vi "RegisterCheck.vi"(8 "error in":errorcluster caption="错误输入", 9 "CMD2":string="AT+CGREG?", 10 "CMD1":string="AT+CREG?", 11 "COMIn":refnum<visa-resource-name>) -> (0 "error out":errorcluster caption="错误输出", 1 "反馈":string, 3 "Result":bool)   [LabVIEW 2013]
uses:
  C:/Program Files/National Instruments/LabVIEW 2013/examples/Instrument IO/Serial/support/Serial - Settings.ctl
  <vilib>/Instr/_visa.llb/VISA Flush IO Buffer Mask.ctl
  <vilib>/Instr/_visa.llb/VISA Configure Serial Port (Instr).vi
panel:
  out "CGREG响应":string
  out "CREG响应":string
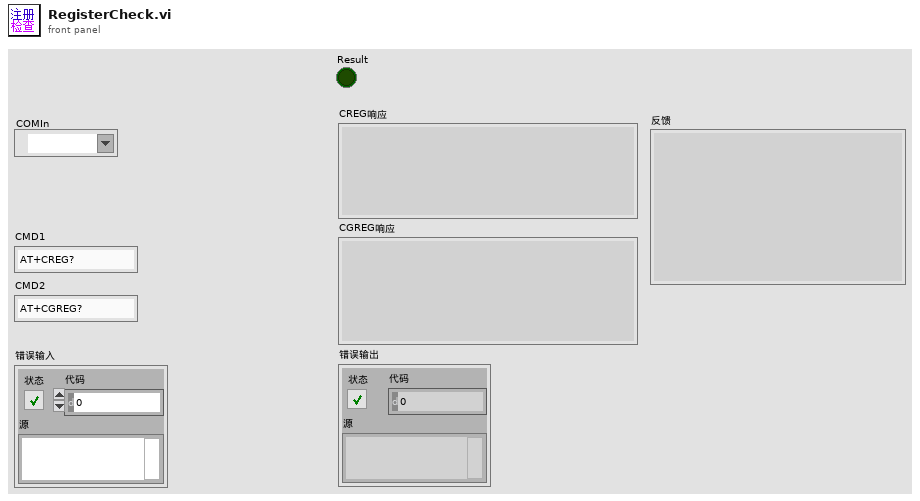
[diagram p1: front panel]
types:
  T1 = typedef "VISA Flush IO Buffer Mask.ctl" = u16
  T2 = typedef "Serial - Settings.ctl" = cluster{"波特率":u32, "数据比特":u16, "奇偶":enum16{"None", "Odd", "Even", "Mark", "Space"}, "停止位":u16, "流控制":u16}
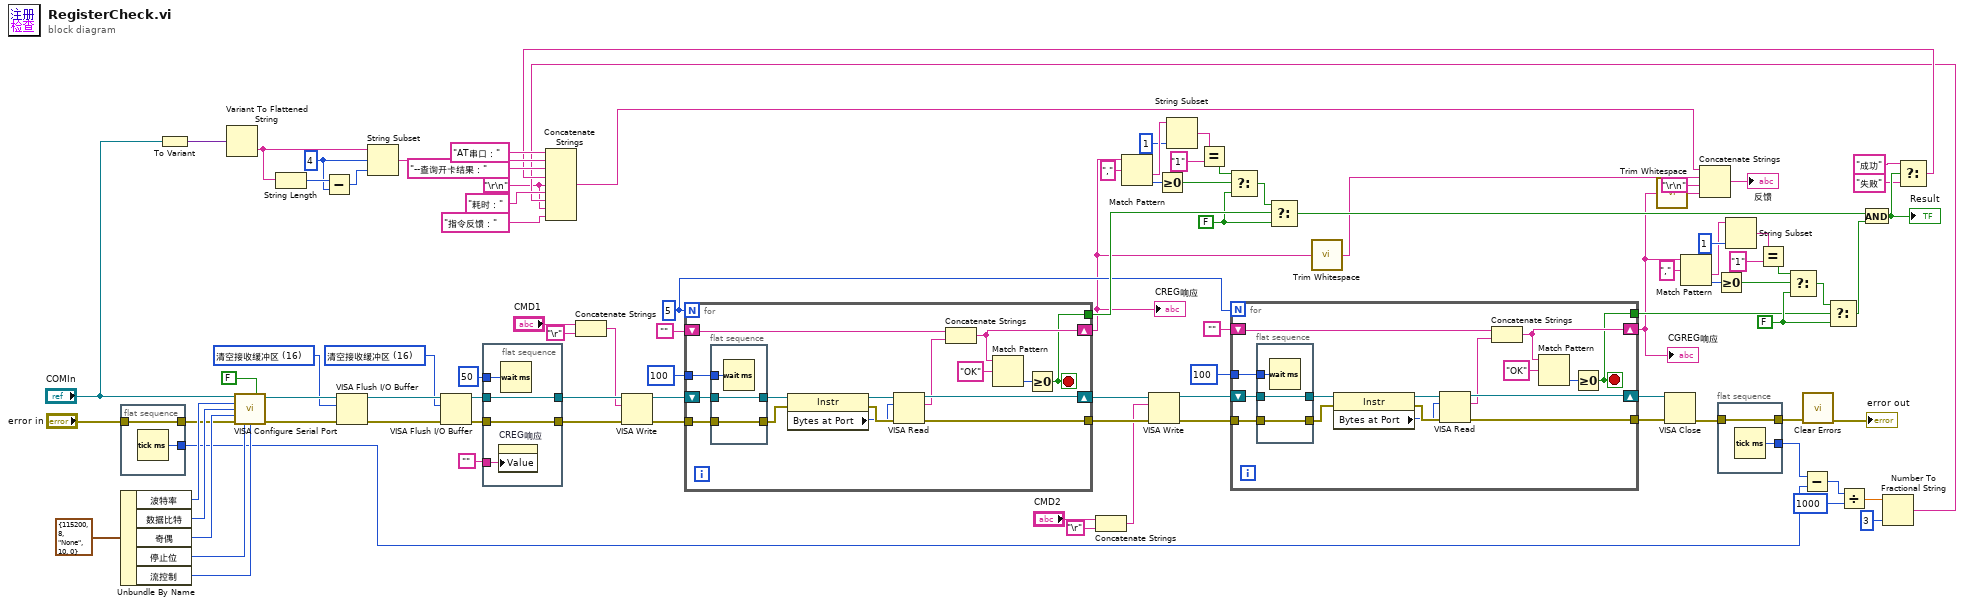
[diagram p0: block diagram]
diagram:
  w3 = "\r\n"
  w24 = 4
  w57 = FALSE
  w61 = FALSE
  w38 = 5
  w85 = T1 16 items=["清空接收缓冲区"=16, "向设备写入传输缓冲区"=32, "清空接收缓冲区（无I/O）"=64, "清空传输缓冲区"=128] ("Mask")
  w88 = T1 16 items=["清空接收缓冲区"=16, "向设备写入传输缓冲区"=32, "清空接收缓冲区（无I/O）"=64, "清空传输缓冲区"=128] ("Mask")
  n1 = flat-sequence {
    tunnel: [w99] -> w15
    tunnel: "error in" -> [w99]
    tunnel: [w98] -> w10
    frame #0 {
      n2 = Tick Count (ms)() -> (millisecond timer value=w98:u32)
    }
  }
  n3 = Unbundle By Name(T2 {"波特率"=115200, "数据比特"=8, "奇偶"=enum."None", "停止位"=10, "流控制"=0} ("串口设置")) -> ("波特率"=w96:u32, "数据比特"=w95:u16, "奇偶"=w94:enum16{"None", "Odd", "Even", "Mark", "Space"}, "停止位"=w93:u16, "流控制"=w92:u16)
  n4 = To Variant(anything="COMIn") -> (Variant=w28:variant)
  n5 = Variant To Flattened String(Variant=w28) -> (data string=w27:string)  [unwired: 1 out]
  n6 = call-poly "VISA Configure Serial Port"("VISA resource name"="COMIn", "Enable Termination\nChar (T)"=FALSE ("Enable Termination\nChar (T)"), "baud rate (9600)"=w96, "data bits (8)"=w95, "parity (0:none)"=w94, "error in (no error)"=w15, "stop bits (10: 1 bit)"=w93, "flow control (0:none)"=w92) -> ("VISA resource name out"=w90:refnum<visa-resource-name>, "error out"=w89:errorcluster)  [unwired: 6 in]
  n7 = String Length(string=w27) -> (length=w26:i32)
  n8 = Subtract(x=w26, y=w24) -> (x-y=w25:i32)
  n9 = VISA Flush I/O Buffer(VISA resource name=w90, mask (16)=w88, error in (no error)=w89) -> (VISA resource name out=w87:refnum<visa-resource-name>, error out=w86:errorcluster)
  n10 = String Subset(string=w27, offset (0)=w24, length (rest)=w25) -> (substring=w23:string)
  n11 = VISA Flush I/O Buffer(VISA resource name=w87, mask (16)=w85, error in (no error)=w86) -> (VISA resource name out=w84:refnum<visa-resource-name>, error out=w83:errorcluster)
  n12 = flat-sequence {
    tunnel: w84 -> [w102]
    tunnel: [w101] -> w80
    tunnel: w83 -> [w101]
    tunnel: 50 -> [w103]
    tunnel: [w102] -> w81
    tunnel: "" -> [w100]
    frame #0 {
      n13 = property on="CREG响应" class="Str"("Value"=w100) -> ()  [unwired: 2 in, 2 out]
      n14 = Wait (ms)(milliseconds to wait=w103) -> ()  [unwired: 1 out]
    }
  }
  n15 = Concatenate Strings("CMD1", "\r") -> (w78:string)
  n16 = VISA Write(VISA resource name=w81, write buffer=w78, error in (no error)=w80) -> (VISA resource name out=w76:refnum<visa-resource-name>, error out=w75:errorcluster)  [unwired: 1 out]
  n17 = for {
    N: w38 -> [_]
    shift-right: [w111] -> w46
    shift-left: w76 -> [w119]
    tunnel: w75 -> [w118]
    tunnel: 100 -> [w117]
    shift-right: [w107] -> w34
    shift-left: "" -> [w110]
    tunnel: [w108] -> w44
    tunnel: [w104] -> w63
    stop <- w104 stop-if-true
    n18 = flat-sequence {
      tunnel: w119 -> [w121]
      tunnel: w118 -> [w120]
      tunnel: w117 -> [w122]
      tunnel: [w121] -> w116
      tunnel: [w120] -> w115
      frame #0 {
        n19 = Wait (ms)(milliseconds to wait=w122) -> ()  [unwired: 1 out]
      }
    }
    n20 = property class="Instr"(reference=w116, error in=w115) -> (reference out=w112:refnum<visa-resource-name>, error out=w114:errorcluster, "Bytes at Port"=w113:u32)
    n21 = VISA Read(VISA resource name=w112, byte count=w113, error in (no error)=w114) -> (VISA resource name out=w111:refnum<visa-resource-name>, read buffer=w109:string, error out=w108:errorcluster)  [unwired: 1 out]
    n22 = Concatenate Strings(w110, w109) -> (w107:string)
    n23 = Match Pattern(string=w107, regular expression="OK" ("正则表达式")) -> (offset past match=w105:i32)  [unwired: 1 in, 3 out]
    n24 = Greater Or Equal To 0?(x=w105) -> (x >= 0?=w104:bool)
  }
  "CREG响应" <- w34
  n25 = Concatenate Strings("CMD2", "\r") -> (w39:string)
  n26 = Match Pattern(string=w34, regular expression="," ("正则表达式")) -> (after substring=w68:string, offset past match=w70:i32)  [unwired: 1 in, 2 out]
  n27 = VISA Write(VISA resource name=w46, write buffer=w39, error in (no error)=w44) -> (VISA resource name out=w45:refnum<visa-resource-name>, error out=w43:errorcluster)  [unwired: 1 out]
  n28 = Greater Or Equal To 0?(x=w70) -> (x >= 0?=w69:bool)
  n29 = String Subset(string=w68, length (rest)=1 ("长度（剩余）")) -> (substring=w66:string)  [unwired: 1 in]
  n30 = Equal?(x=w66, y="1") -> (x = y?=w64:bool)
  n31 = Select(t=w64, s=w69, f=w61) -> (s? t:f=w62:bool)
  n32 = for {
    N: w38 -> [_]
    shift-right: [w130] -> w60
    shift-left: w45 -> [w138]
    tunnel: w43 -> [w137]
    tunnel: 100 -> [w136]
    shift-right: [w126] -> w35
    shift-left: "" -> [w129]
    tunnel: [w127] -> w59
    tunnel: [w123] -> w47
    stop <- w123 stop-if-true
    n33 = flat-sequence {
      tunnel: w138 -> [w140]
      tunnel: w137 -> [w139]
      tunnel: w136 -> [w141]
      tunnel: [w140] -> w135
      tunnel: [w139] -> w134
      frame #0 {
        n34 = Wait (ms)(milliseconds to wait=w141) -> ()  [unwired: 1 out]
      }
    }
    n35 = property class="Instr"(reference=w135, error in=w134) -> (reference out=w131:refnum<visa-resource-name>, error out=w133:errorcluster, "Bytes at Port"=w132:u32)
    n36 = VISA Read(VISA resource name=w131, byte count=w132, error in (no error)=w133) -> (VISA resource name out=w130:refnum<visa-resource-name>, read buffer=w128:string, error out=w127:errorcluster)  [unwired: 1 out]
    n37 = Concatenate Strings(w129, w128) -> (w126:string)
    n38 = Match Pattern(string=w126, regular expression="OK" ("正则表达式")) -> (offset past match=w124:i32)  [unwired: 1 in, 3 out]
    n39 = Greater Or Equal To 0?(x=w124) -> (x >= 0?=w123:bool)
  }
  "CGREG响应" <- w35
  n40 = Select(t=w62, s=w63, f=w61) -> (s? t:f=w37:bool)
  n41 = call <vilib>:"Trim Whitespace.vi"("string"=w34) -> ("trimmed string"=w33:string)  [unwired: 1 in]
  n42 = call <vilib>:"Trim Whitespace.vi"("string"=w35) -> ("trimmed string"=w31:string)  [unwired: 1 in]
  n43 = VISA Close(VISA resource name=w60, error in (no error)=w59) -> (error out=w13:errorcluster)
  n44 = Match Pattern(string=w35, regular expression="," ("正则表达式")) -> (after substring=w51:string, offset past match=w49:i32)  [unwired: 1 in, 2 out]
  n45 = Greater Or Equal To 0?(x=w49) -> (x >= 0?=w50:bool)
  n46 = flat-sequence {
    tunnel: [w143] -> w12
    tunnel: w13 -> [w143]
    tunnel: [w142] -> w11
    frame #0 {
      n47 = Tick Count (ms)() -> (millisecond timer value=w142:u32)
    }
  }
  n48 = String Subset(string=w51, length (rest)=1 ("长度（剩余）")) -> (substring=w53:string)  [unwired: 1 in]
  n49 = Equal?(x=w53, y="1") -> (x = y?=w55:bool)
  n50 = Select(t=w55, s=w50, f=w57) -> (s? t:f=w56:bool)
  n51 = Subtract(x=w11, y=w10) -> (x-y=w9:u32)
  n52 = call <vilib>:"Clear Errors.vi"("error in (no error)"=w12) -> ("error out"=→"error out":errorcluster)  [unwired: 6 in]
  n53 = Select(t=w56, s=w47, f=w57) -> (s? t:f=w36:bool)
  n54 = Divide(x=w9, y=u32 1000) -> (x/y=w7:dbl)
  n55 = And(x=w37, y=w36) -> (x .and. y?=w20:bool)
  "Result" <- w20
  n56 = Number To Fractional String(number=w7, precision (6)=i16 3 ("精度(6)")) -> (F-format string=w4:string)  [unwired: 2 in]
  n57 = Select(t="成功" ("反馈 2"), s=w20, f="失败" ("反馈 2")) -> (s? t:f=w16:string)
  n58 = Concatenate Strings("AT串口：" ("字符串"), w23, "--查询开卡结果：" ("字符串"), w16, w3, "耗时：" ("字符串"), w4, w3, "指令反馈：" ("字符串")) -> (w21:string)
  n59 = Concatenate Strings(w21, w33, "\r\n", w31) -> (→"反馈":string)
